vi "Project Save for Previous.vi"(7 "LabVIEW Previous Version":T1=enum."2015", 8 "Error In":errorcluster) -> (0 "Error Out":errorcluster, 3 "Destination":path)   [LabVIEW 2017, in "Scripts.lvlib"]
doc: "Saves a project to a previous version of LabVIEW. The output is saved to \"<project root>\\target\\<Target Version>\", where \"<project root>\" is the folder that contains the LabVIEW project file (.lvproj) and \"<Target Version>\" is the previous version of LabVIEW, such as \"15.0\" for LabVIEW 2015."
uses:
  Scripts.lvlib
  LabVIEW Versions.ctl
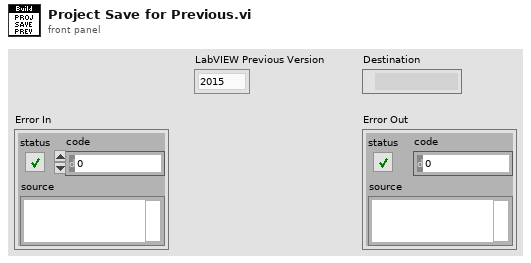
[diagram p1: front panel]
types:
  T1 = typedef "Scripts.lvlib/LabVIEW Versions.ctl" = enum16{"2009", "2010", "2011", "2012", "2013", "2014", "2015", "2016", "2017", "2018"}
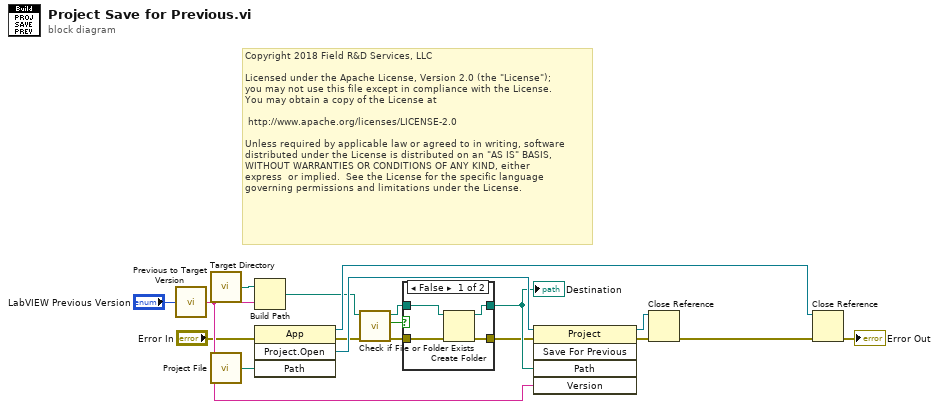
[diagram p0: block diagram]
diagram:
  # "Copyright 2018 Field R&D Services, LLC\n\nLicensed under the Apache License, Version 2.0 (the \"License\");\nyou may not use this file except in compliance with the License.\nYou may obtain a copy of the License at\n\n\thttp://www.apache.org/licenses/LICENSE-2.0\n\nUnless required by applicable law or agreed to in writing, software\ndistributed under the License is distributed on an \"AS IS\" BASIS,\nWITHOUT WARRANTIES OR CONDITIONS OF ANY KIND, either \nexpress  or implied.  See the License for the specific language \ngoverning permissions and limitations under the License."
  n1 = call "Previous to Target Version.vi"("Previous Version"="LabVIEW Previous Version") -> ("Target Version"=w4:string)
  n2 = call "Target Directory.vi"() -> ("Target Directory"=w1:path)
  n3 = call "Project File.vi"() -> ("Project File"=w2:path)
  n4 = Build Path(base path=w1, name or relative path=w4) -> (appended path=w5:path)
  n5 = invoke class="App" method="Project.Open"(error in="Error In", "Path"=w2) -> (reference out=w15:refnum<vi>, error out=w12:errorcluster, "Project:Open"=w18:refnum<vi>)  [unwired: 2 in, 1 out]
  n6 = call <vilib>:"Check if File or Folder Exists.vi"("error in (no error)"=w12, "path"=w5) -> ("error out"=w8:errorcluster, "file or folder exists?"=w11:bool, "dup path"=w10:path)  [unwired: 7 in]
  n7 = case shown="False" w11 {
    tunnel: w10 -> [w22 w24]
    tunnel: [w19 w24] -> w9
    tunnel: w8 -> [w21 w23]
    tunnel: [w20 w23] -> w7
    frame False {
      n8 = Create Folder(path (use dialog)=w22, error in=w21) -> (created path=w19:path, error out=w20:errorcluster)  [unwired: 1 in, 1 out]
    }
    frame True {
    }
  }
  "Destination" <- w9
  n9 = invoke class="Project" method="Save For Previous"(reference=w18, error in=w7, "Path"=w9, "Version"=w4) -> (reference out=w16:refnum<vi>, error out=w17:errorcluster)  [unwired: 1 in, 3 out]
  n10 = Close Reference(reference=w16, error in (no error)=w17) -> (error out=w14:errorcluster)
  n11 = Close Reference(reference=w15, error in (no error)=w14) -> (error out=→"Error Out":errorcluster)
